vi "FF_determine_addressing_changes_required.vi"(2 "pdTag list":string[](array[string]), 3 "FF address list":string[](array[string])) -> (0 "need to display\nmessage?":bool, 1 "Result":string)   [LabVIEW 2016]
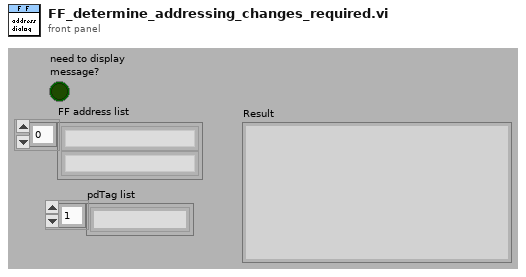
[diagram p1: front panel]
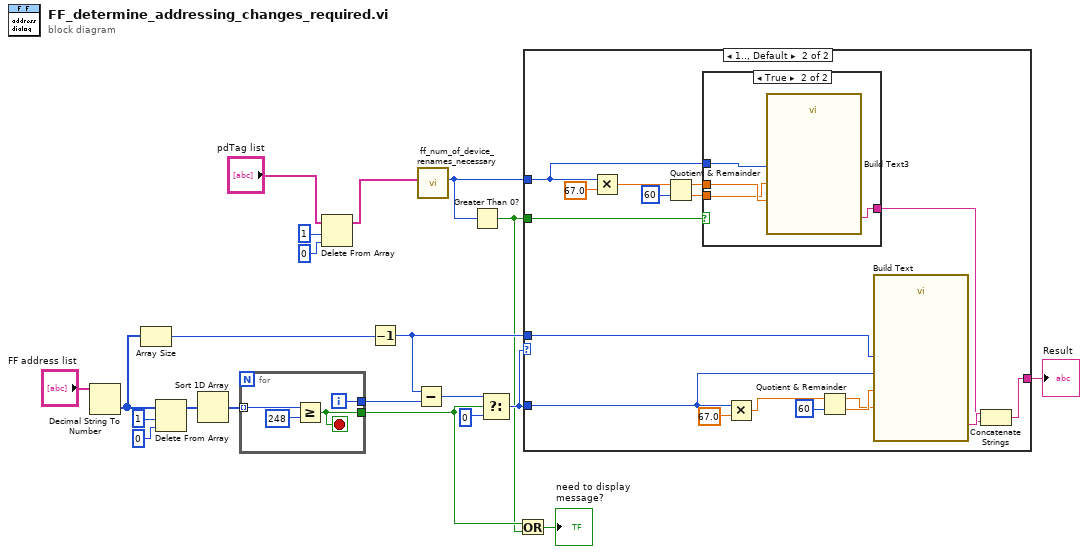
[diagram p0: block diagram]
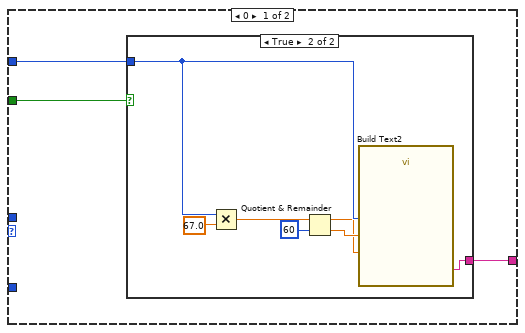
[diagram p2: hidden frame]
diagram:
  n1 = Decimal String To Number(string="FF address list") -> (number=w16:i32[])  [unwired: 2 in, 1 out]
  n2 = Array Size(array=w16) -> (size(s)=w20:i32)
  n3 = Delete From Array(array=w16, length=1, index=0) -> (array with subset deleted=w13:i32[])  [unwired: 1 out]
  n4 = Sort 1D Array(array=w13) -> (sorted array=w21:i32[])
  n5 = for {
    tunnel: w21 -> [w25] mode=indexing
    tunnel: [w23] -> w7
    tunnel: [w22] -> w18
    i -> [w22]
    stop <- w23 stop-if-true
    n6 = Greater Or Equal?(x=w25, y=248) -> (x >= y?=w23:bool)
  }
  n7 = Delete From Array(array="pdTag list", length=1, index=0) -> (array with subset deleted=w1:string[])  [unwired: 1 out]
  n8 = Decrement(x=w20) -> (x-1=w19:i32)
  n9 = Subtract(x=w19, y=w18) -> (x-y=w12:i32)
  n10 = call "ff_num_of_device_renames_necessary.vi"("pdTag list"=w1) -> ("num of renames necessary"=w8:i32)  [unwired: 10 in]
  n11 = Greater Than 0?(x=w8) -> (x > 0?=w6:bool)
  n12 = Select(t=w12, s=w7, f=0) -> (s? t:f=w10:i32)
  n13 = Or(x=w7, y=w6) -> (x .or. y?=→"need to display\nmessage?":bool)
  n14 = case shown="1.., Default" w10 {
    tunnel: w19 -> [_ w52]
    tunnel: w10 -> [_ w50]
    tunnel: [w27 w43] -> w17
    tunnel: w6 -> [w26 w44]
    tunnel: w8 -> [w28 w38]
    frame 0 {
      n15 = case shown="True" w26 {
        tunnel: w28 -> [_ w32]
        tunnel: [_ w29] -> w27
        frame False {
        }
        frame True {
          n16 = Multiply(x=w32, y=67.0) -> (x*y=w34:dbl)
          n17 = Quotient & Remainder(x=w34, y=60) -> (x-y*floor(x/y)=w30:dbl, floor(x/y)=w31:dbl)
          n18 = call "Build Text2"("num devices"=w32, "min"=w31, "sec"=w30) -> ("Result"=w29:string)  [unwired: 11 in, 1 out]
        }
      }
    }
    frame 1.., Default {
      n19 = Multiply(x=w38, y=67.0) -> (x*y=w40:dbl)
      n20 = Quotient & Remainder(x=w40, y=60) -> (x-y*floor(x/y)=w37:dbl, floor(x/y)=w36:dbl)
      n21 = case shown="True" w44 {
        tunnel: w38 -> [_ w56]
        tunnel: [_ w55] -> w42
        tunnel: w37 -> [_ w54]
        tunnel: w36 -> [_ w53]
        frame False {
        }
        frame True {
          n22 = call "Build Text3"("num devices"=w56, "min"=w53, "sec"=w54) -> ("Result"=w55:string)  [unwired: 11 in, 1 out]
        }
      }
      n23 = Multiply(x=w50, y=67.0) -> (x*y=w48:dbl)
      n24 = Quotient & Remainder(x=w48, y=60) -> (x-y*floor(x/y)=w45:dbl, floor(x/y)=w46:dbl)
      n25 = call "Build Text"("seconds"=w45, "total number"=w52, "num in default"=w50, "minutes"=w46) -> ("Result"=w51:string)  [unwired: 10 in, 1 out]
      n26 = Concatenate Strings(w51, w42) -> (w43:string)
    }
  }
  "Result" <- w17
